vi "spec_SetGrating.vi"(8 "error in (no error)":errorcluster, 10 "GratingSelected":string, 11 "LightField Automation in":refnum<class "LightField Automation.lvclass">) -> (0 "error out":errorcluster, 3 "LightField Automation out":refnum<class "LightField Automation.lvclass">)   [LabVIEW 2020, in "LightField Automation.lvclass"]
uses:
  LightField Automation.lvclass
  C:/Program Files/Princeton Instruments/LightField/PrincetonInstruments.LightFieldAddInSupportServices.dll
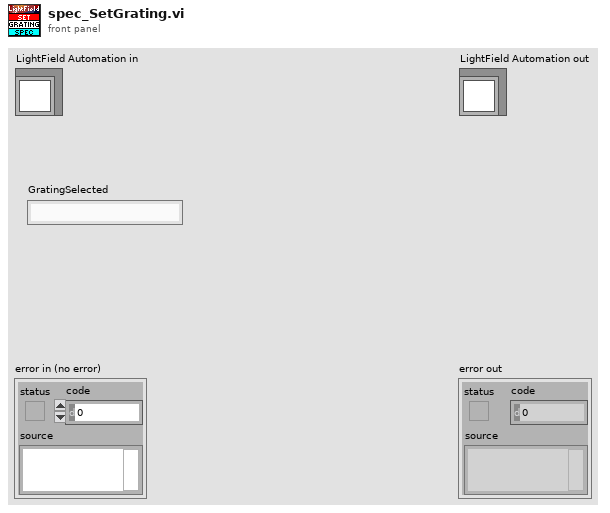
[diagram p1: front panel]
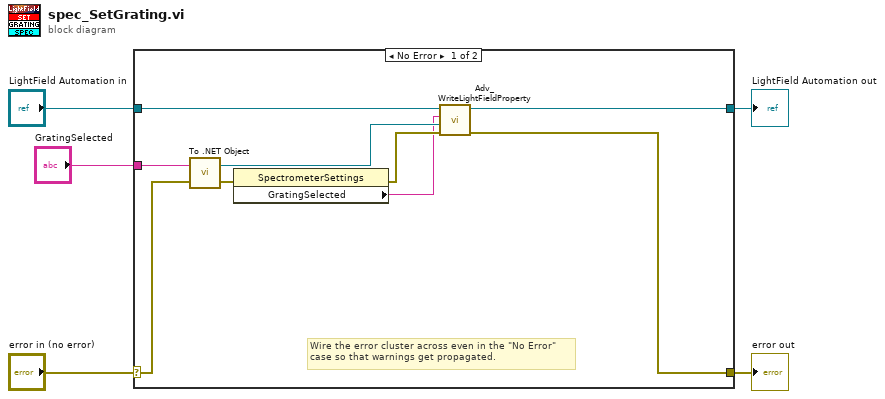
[diagram p0: block diagram]
diagram:
  n1 = case shown="No Error" "error in (no error)" {
    selector: "error in (no error)" -> [w12 w16]
    tunnel: [w7 w16] -> w4
    tunnel: [w6 w15] -> w2
    tunnel: "LightField Automation in" -> [w14 w15]
    tunnel: "GratingSelected" -> [w13 _]
    frame No Error {
      # "Wire the error cluster across even in the \"No Error\"\ncase so that warnings get propagated."
      n2 = call <vilib>:"To .NET Object.vi"("error in (no error)"=w12, "anything"=w13) -> ("error out"=w10:errorcluster, ".NET object"=w11:refnum<k24>)
      n3 = property class="SpectrometerSettings"(error in=w10) -> (error out=w9:errorcluster, "GratingSelected"=w8:string)  [unwired: 1 in, 1 out]
      n4 = call "Adv_WriteLightFieldProperty.vi"("error in (no error)"=w9, "value"=w11, "setting"=w8, "LightField Automation in"=w14) -> ("error out"=w7:errorcluster, "LightField Automation out"=w6:refnum<class "LightField Automation.lvclass">)  [unwired: 6 in]
    }
    frame Error {
    }
  }
  "error out" <- w4
  "LightField Automation out" <- w2
